vi "Get Resource by RID.vi"(8 "error in (no error)":errorcluster, 10 "RID":string, 11 "LangFile in":refnum<class "Resource Data.lvclass">) -> (0 "error out":errorcluster, 1 "Found?":bool, 2 "Resource":T1, 3 "LangFile out":refnum<class "Resource Data.lvclass">, 5 "Index":i32)   [LabVIEW 2013, in "SET Project Data.lvlib" / "Resource Data.lvclass"]
uses:
  Resource Data.lvclass
  Types/ProjFile_Resource Entry.ctl
  Resource Data.lvclass/Resource Data.ctl
  SET Project Data.lvlib
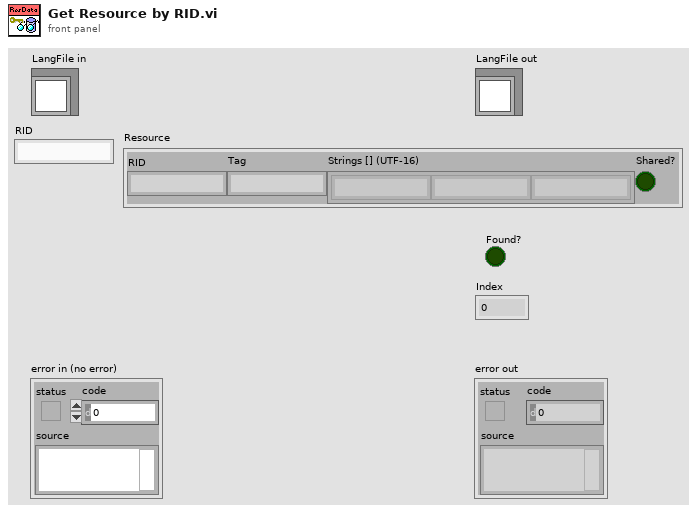
[diagram p1: front panel]
types:
  T1 = typedef "SET Project Data.lvlib/ProjFile_Resource Entry.ctl" = cluster{"RID":string, "Tag":string, "Strings [] (UTF-16)":string[], "Shared?":bool}
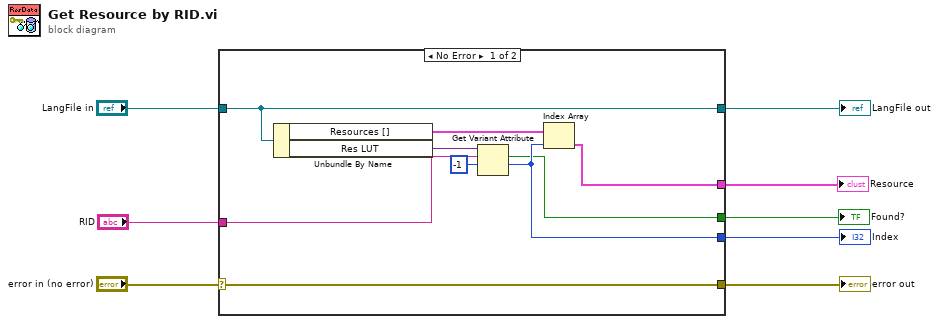
[diagram p0: block diagram]
diagram:
  n1 = case shown="No Error" "error in (no error)" {
    selector: "error in (no error)" -> [w17 w19]
    tunnel: [w17 w19] -> w7
    tunnel: [w16 w18] -> w5
    tunnel: "LangFile in" -> [w16 w18]
    tunnel: "RID" -> [w14 _]
    tunnel: [w10 _] -> w3
    tunnel: [w9 _] -> w2
    tunnel: [w11 _] -> w1
    frame No Error {
      n2 = Unbundle By Name(w16) -> ("Resources []"=w12:T1[], "Res LUT"=w15:variant)
      n3 = Get Variant Attribute(Variant=w15, name=w14, default value (empty Variant)=-1) -> (found=w10:bool, value=w11:i32)  [unwired: 1 in, 2 out]
      n4 = Index Array(array=w12, index=w11) -> (element=w9:T1)
    }
    frame Error {
    }
  }
  "error out" <- w7
  "LangFile out" <- w5
  "Found?" <- w3
  "Resource" <- w2
  "Index" <- w1
